vi "Main Page.vi"(8 "error in (no error)":errorcluster, 11 "Node Ptr":T1 format="%.0x") -> (0 "error out":errorcluster)   [LabVIEW 2027, in "Embedded Data Logger System Explorer.lvlib"]
uses:
  Embedded Data Logger System Explorer.lvlib
  <vilib>/NI VeriStand/Custom Device API/Custom Device Item Ref.ctl
  <vilib>/NI VeriStand/Custom Device API/Custom Device API.lvlib
  Scripting/Embedded Data Logger Scripting.lvlib
panel:
  in  "Header 2":cluster{"Section Name":string}={"Section Name"="TDMS Data Log Files"}
  in  "Remove":bool
  in  "TDMS Log Files":i32(listbox)
  in  "FIFO Depth":i32=100
  in  "Add File":bool
  in  "Header":cluster{"Section Name":string}={"Section Name"="Embedded Data Logger Settings"}
  in  "Name":string
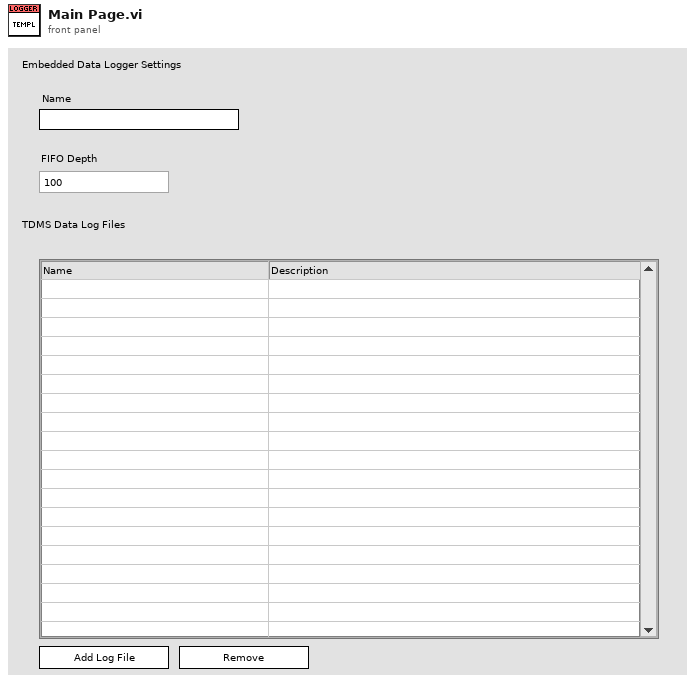
[diagram p1: front panel]
types:
  T1 = typedef "Custom Device API.lvlib/Custom Device Item Ref.ctl" = u64
  T2 = typedef "Custom Device API.lvlib/Custom Device Item Info.ctl" = cluster{"Name":string, "Is Channel":bool, "GUID":string, "Is Waveform":bool}
  T3 = typedef "Custom Device API.lvlib/Custom Device Commands.ctl" = enum16{"Default", "Item renamed", "Shutdown", "Dynamic button pressed"}
  T4 = typedef "LVRowAndColumnTypeDef.ctl" = cluster{"Row":i32, "Column":i32}
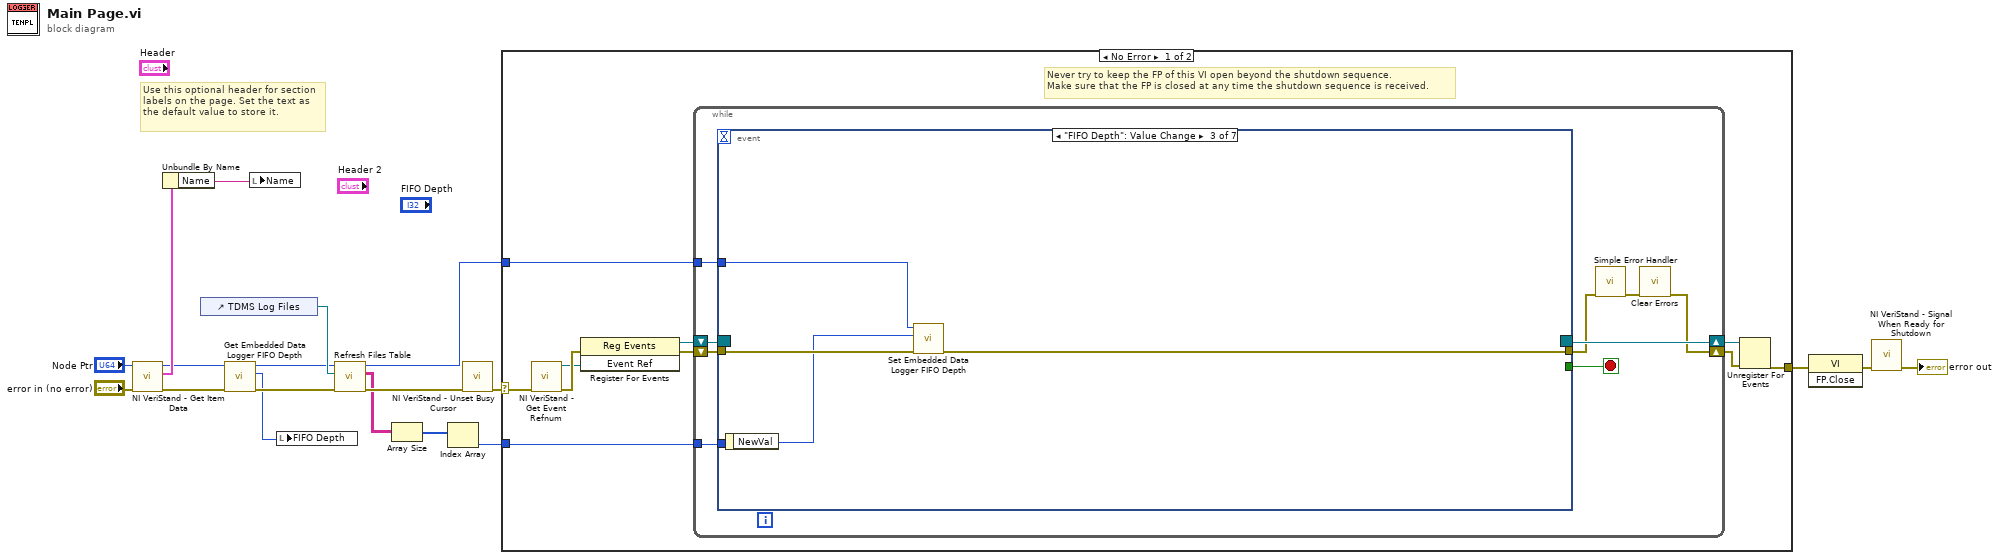
[diagram p0: block diagram]
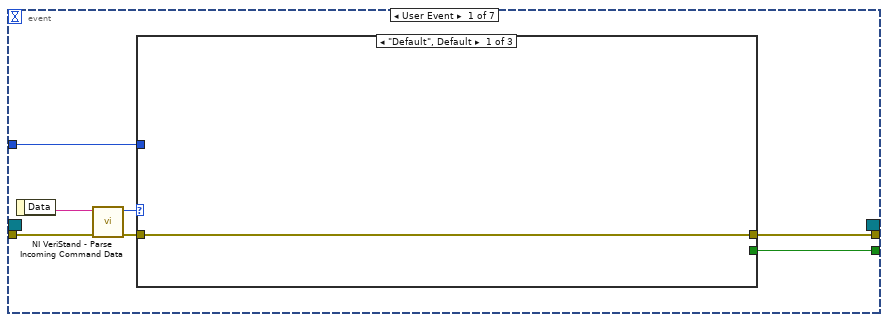
[diagram p2: hidden frame]
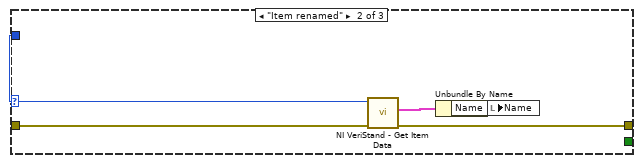
[diagram p3: hidden frame]
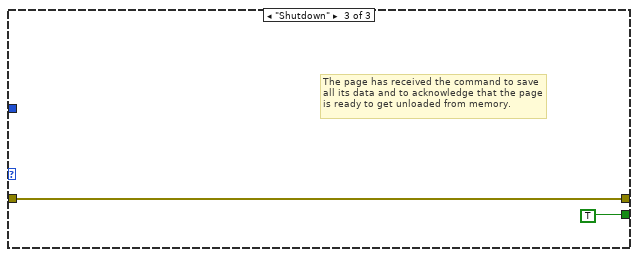
[diagram p4: hidden frame]
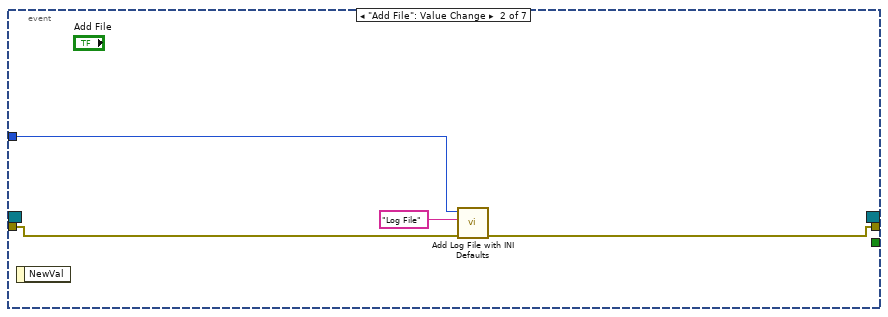
[diagram p5: hidden frame]
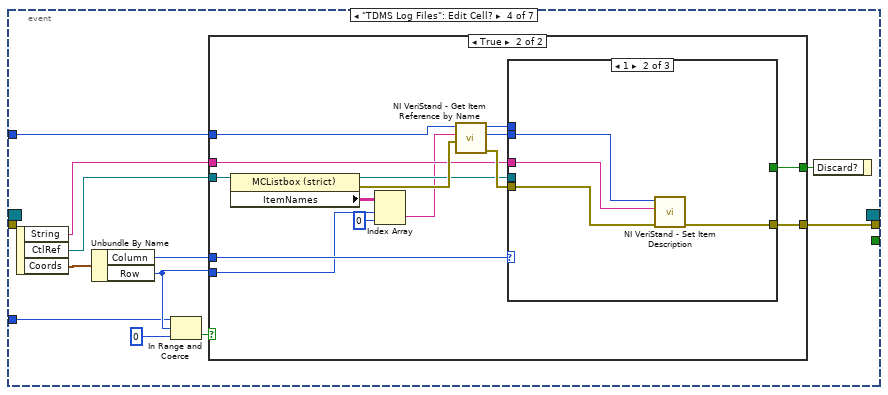
[diagram p6: hidden frame]
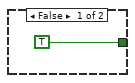
[diagram p7: hidden frame]
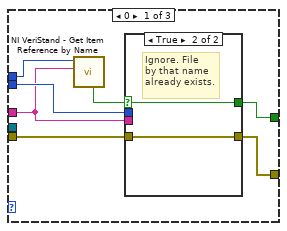
[diagram p8: hidden frame]
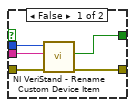
[diagram p9: hidden frame]
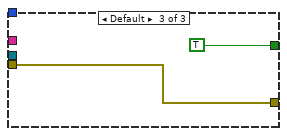
[diagram p10: hidden frame]
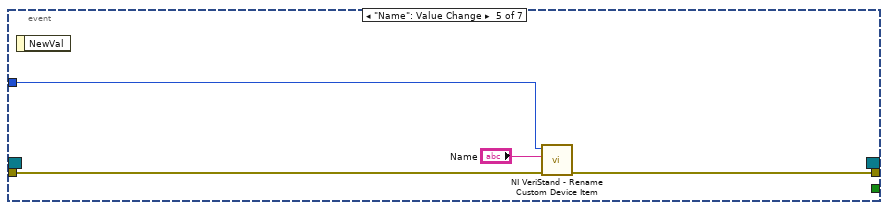
[diagram p11: hidden frame]
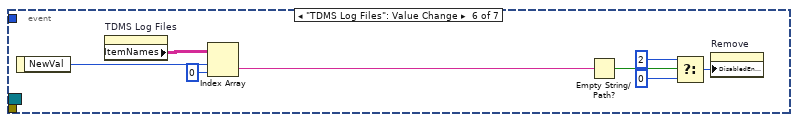
[diagram p12: hidden frame]
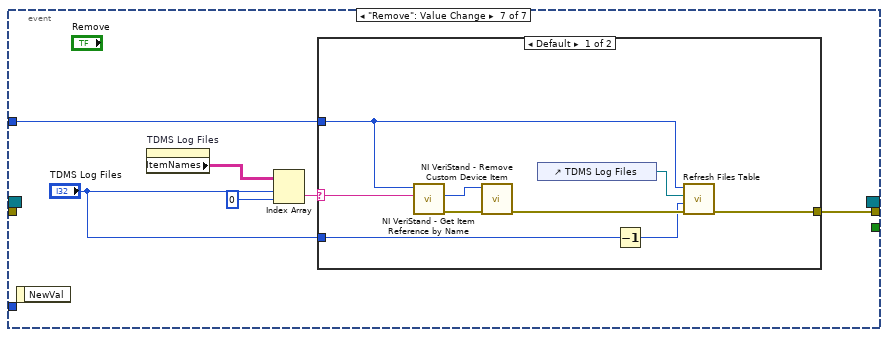
[diagram p13: hidden frame]
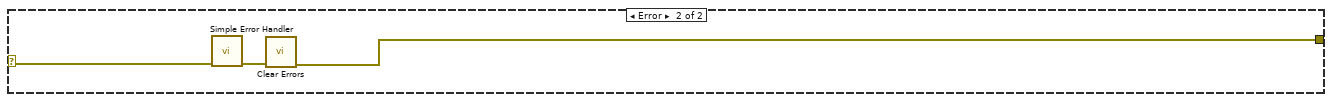
[diagram p15: hidden frame]
diagram:
  # "Use this optional header for section labels on the page. Set the text as the default value to store it."
  n1 = call <vilib>:"NI VeriStand - Get Item Data.vi"("error in (no error)"="error in (no error)", "Item Ref in"="Node Ptr") -> ("error out"=w12:errorcluster, "Item Info"=w14:T2, "Item Ref out"=w11:T1)  [unwired: 7 out]
  n2 = Unbundle By Name(w14) -> ("Name"=w13:string)
  n3 = control-ref of="TDMS Log Files"() -> (w2:refnum<vi>)
  n4 = call "Get Embedded Data Logger FIFO Depth.vi"("error in"=w12, "embedded data logger in"=w11) -> ("error out"=w19:errorcluster, "fifo depth"=w10:i32, "embedded data logger out"=w1:T1)  [unwired: 7 in]
  n5 = local write "Name"(w13) -> ()
  n6 = local write "FIFO Depth"(w10) -> ()
  n7 = call "Refresh Files Table.vi"("error in (no error)"=w19, "MulticolumnListbox in"=w2, "Section Ref in"=w1) -> ("error out"=w9:errorcluster, "Array"=w8:string[][], "Section Ref out"=w5:T1)  [unwired: 6 in]
  n8 = Array Size(array=w8) -> (size(s)=w7:i32[])
  n9 = Index Array(array=w7) -> (element=w6:i32)  [unwired: 1 in]
  n10 = call <vilib>:"NI VeriStand - Unset Busy Cursor.vi"("error in (no error)"=w9) -> ("error out"=w15:errorcluster)  [unwired: 10 out]
  n11 = case shown="No Error" w15 {
    selector: w15 -> [w21 w138]
    tunnel: [w26 w136] -> w18
    tunnel: w5 -> [w22 _]
    tunnel: w6 -> [w20 _]
    frame No Error {
      # "Never try to keep the FP of this VI open beyond the shutdown sequence.\nMake sure that the FP is closed at any time the shutdown sequence is received."
      n12 = call <vilib>:"NI VeriStand - Get Event Refnum.vi"("error in (no error)"=w21) -> ("error out"=w29:errorcluster, "Event Ref"=w25:refnum<user-event>)  [unwired: 9 out]
      n13 = register-events(error in=w29, w25) -> (reference out=w23:refnum<event-registration>, error out=w24:errorcluster)  [unwired: 1 in]
      n14 = while {
        tunnel: w22 -> [w34]
        shift-right: [w31] -> w27
        shift-left: w24 -> [w37]
        shift-right: [w38] -> w28
        shift-left: w23 -> [w36]
        tunnel: w20 -> [w30]
        stop <- w35 stop-if-true
        n15 = event shown="[2] \"FIFO Depth\": Value Change" {
          selector: w36 -> [_ _ _ _ _ _ _]
          dyn-events: [_ _ _ _ _ _ _] -> w38
          timeout: _ -> [_ _ _ _ _ _ _]
          tunnel: w37 -> [w45 w56 w61 _ w112 _ _]
          tunnel: [w41 _ _ _ _ _ _] -> w35
          tunnel: [w40 w54 w58 w68 w111 _ w123] -> w33
          tunnel: w34 -> [w39 w55 w60 w63 w110 _ w124]
          tunnel: w30 -> [_ _ _ w62 _ _ _]
          event User Event {
            n16 = event-data() -> ("Data"=w44:string)  [unwired: 1 out]
            n17 = call <vilib>:"NI VeriStand - Parse Incoming Command Data.vi"("error in (no error)"=w45, "Incoming data"=w44) -> ("error out"=w43:errorcluster, "Action"=w42:T3)  [unwired: 8 out]
            n18 = case shown="\"Default\", Default" w42 {
              tunnel: w43 -> [w46 w51 w52]
              tunnel: [_ _ TRUE] -> w41
              tunnel: [w46 w48 w52] -> w40
              tunnel: w39 -> [_ w50 _]
              frame "Default", Default {
              }
              frame "Item renamed" {
                n19 = call <vilib>:"NI VeriStand - Get Item Data.vi"("error in (no error)"=w51, "Item Ref in"=w50) -> ("error out"=w48:errorcluster, "Item Info"=w49:T2)  [unwired: 8 out]
                n20 = Unbundle By Name(w49) -> ("Name"=w47:string)
                n21 = local write "Name"(w47) -> ()
              }
              frame "Shutdown" {
                # "The page has received the command to save all its data and to acknowledge that the page is ready to get unloaded from memory."
              }
            }
          }
          event "Add File": Value Change {
            n22 = event-data() -> ()  [unwired: 2 out]
            n23 = call "Add Log File with INI Defaults.vi"("error in"=w56, "log file name"="Log File" ("Default Name"), "embedded data logger in"=w55) -> ("error out"=w54:errorcluster)  [unwired: 6 in, 2 out]
          }
          event "FIFO Depth": Value Change {
            n24 = event-data() -> ("NewVal"=w59:i32)  [unwired: 1 out]
            n25 = call "Set Embedded Data Logger FIFO Depth.vi"("error in"=w61, "fifo depth"=w59, "embedded data logger in"=w60) -> ("error out"=w58:errorcluster)  [unwired: 7 in, 1 out]
          }
          event "TDMS Log Files": Edit Cell? {
            n26 = event-data() -> ("String"=w65:string, "CtlRef"=w64:refnum<vi>, "Coords"=w66:T4)  [unwired: 1 out]
            n27 = Unbundle By Name(w66) -> ("Column"=w72:i32, "Row"=w70:i32)
            n28 = In Range and Coerce(upper limit=w62, x=w70, lower limit=0) -> (In Range?=w69:bool)  [unwired: 1 out]
            n29 = case shown="True" w69 {
              tunnel: w64 -> [_ w86]
              tunnel: [TRUE w83] -> w67
              tunnel: w65 -> [_ w81]
              tunnel: w63 -> [_ w79]
              tunnel: w70 -> [_ w78]
              tunnel: w72 -> [_ w84]
              tunnel: [_ w80] -> w68
              frame False {
              }
              frame True {
                n30 = property class="MCListbox (strict)"(reference=w86) -> (reference out=w82:refnum<vi>, error out=w88:errorcluster, "ItemNames"=w85:string[][])  [unwired: 1 in]
                n31 = Index Array(array=w85, index (row)=w78, index (col)=0 ("disabled index (col)")) -> (element=w76:string)
                n32 = call <vilib>:"NI VeriStand - Get Item Reference by Name.vi"("error in (no error)"=w88, "Item Name"=w76, "Parent Ref in"=w79) -> ("error out"=w87:errorcluster, "Item Ref"=w75:T1, "Parent Ref out"=w74:T1)  [unwired: 5 in, 1 out]
                n33 = case shown="1" w84 {
                  tunnel: [w89 _ TRUE] -> w83
                  tunnel: w75 -> [w94 w105 _]
                  tunnel: w87 -> [w95 w103 w107]
                  tunnel: w82 -> [_ _ _]
                  tunnel: w81 -> [w91 w104 _]
                  tunnel: [w93 w106 w107] -> w80
                  tunnel: w74 -> [w92 _ _]
                  frame 0 {
                    n34 = call <vilib>:"NI VeriStand - Get Item Reference by Name.vi"("Item Name"=w91, "Parent Ref in"=w92) -> ("Found"=w90:bool)  [unwired: 6 in, 3 out]
                    n35 = case shown="True" w90 {
                      selector: w90 -> [_ w101]
                      tunnel: w95 -> [w100 w102]
                      tunnel: w94 -> [w99 _]
                      tunnel: [w98 w102] -> w93
                      tunnel: w91 -> [w97 _]
                      tunnel: [w96 w101] -> w89
                      frame False {
                        n36 = call <vilib>:"NI VeriStand - Rename Custom Device Item.vi"("error in (no error)"=w100, "New Name"=w97, "Item Ref in"=w99) -> ("error out"=w98:errorcluster, "Request invalid?"=w96:bool)  [unwired: 6 in, 1 out]
                      }
                      frame True {
                        # "Ignore. File\nby that name\nalready exists."
                      }
                    }
                  }
                  frame 1 {
                    n37 = call <vilib>:"NI VeriStand - Set Item Description.vi"("error in (no error)"=w103, "Description"=w104, "Item Ref in"=w105) -> ("error out"=w106:errorcluster)  [unwired: 6 in, 2 out]
                  }
                  frame Default {
                  }
                }
              }
            }
            n38 = event-data("Discard?"=w67) -> ()  [unwired: 1 in, 1 out]
          }
          event "Name": Value Change {
            n39 = event-data() -> ()  [unwired: 2 out]
            n40 = call <vilib>:"NI VeriStand - Rename Custom Device Item.vi"("error in (no error)"=w112, "New Name"="Name", "Item Ref in"=w110) -> ("error out"=w111:errorcluster)  [unwired: 1 in, 7 out]
          }
          event "TDMS Log Files": Value Change {
            n41 = event-data() -> ("NewVal"=w113:i32)  [unwired: 1 out]
            n42 = property on="TDMS Log Files" class="MCListbox (strict)"() -> ("ItemNames"=w114:string[][])  [unwired: 2 in, 2 out]
            n43 = Index Array(array=w114, index (row)=w113, index (col)=0 ("disabled index (col)")) -> (element=w117:string)
            n44 = Empty String/Path?(string/path=w117) -> (empty?=w116:bool)
            n45 = Select(t=u8 2, s=w116, f=u8 0) -> (s? t:f=w118:u8)
            n46 = property on="Remove" class="Bool"("DisabledEnum"=w118) -> ()  [unwired: 2 in, 2 out]
          }
          event "Remove": Value Change {
            n47 = event-data() -> ()  [unwired: 2 out]
            n48 = property on="TDMS Log Files" class="MCListbox (strict)"() -> ("ItemNames"=w122:string[][])  [unwired: 2 in, 2 out]
            n49 = Index Array(array=w122, index (row)="TDMS Log Files", index (col)=0 ("disabled index (col)")) -> (element=w126:string)
            n50 = case shown="Default" w126 {
              selector: w126 -> [w134 _]
              tunnel: w124 -> [w129 _]
              tunnel: [w130 _] -> w123
              tunnel: "TDMS Log Files" -> [w127 _]
              frame Default {
                n51 = call <vilib>:"NI VeriStand - Get Item Reference by Name.vi"("Item Name"=w134, "Parent Ref in"=w129) -> ("error out"=w135:errorcluster, "Item Ref"=w133:T1)  [unwired: 6 in, 2 out]
                n52 = call <vilib>:"NI VeriStand - Remove Custom Device Item.vi"("error in (no error)"=w135, "Item Ref in"=w133) -> ("error out"=w131:errorcluster)  [unwired: 8 in, 1 out]
                n53 = control-ref of="TDMS Log Files"() -> (w132:refnum<vi>)
                n54 = Decrement(x=w127) -> (x-1=w128:i32)
                n55 = call "Refresh Files Table.vi"("error in (no error)"=w131, "Index"=w128, "MulticolumnListbox in"=w132, "Section Ref in"=w129) -> ("error out"=w130:errorcluster)  [unwired: 5 in, 2 out]
              }
              frame "" {
              }
            }
          }
        }
        n56 = call <vilib>:"Simple Error Handler.vi"("error in (no error)"=w33) -> ("error out"=w32:errorcluster)  [unwired: 1 in, 7 out]
        n57 = call <vilib>:"Clear Errors.vi"("error in (no error)"=w32) -> ("error out"=w31:errorcluster)  [unwired: 1 in, 5 out]
      }
      n58 = Unregister For Events(event registration refnum=w28, error in=w27) -> (error out=w26:errorcluster)
    }
    frame Error {
      n59 = call <vilib>:"Simple Error Handler.vi"("error in (no error)"=w138) -> ("error out"=w137:errorcluster)  [unwired: 1 in, 7 out]
      n60 = call <vilib>:"Clear Errors.vi"("error in (no error)"=w137) -> ("error out"=w136:errorcluster)  [unwired: 1 in, 5 out]
    }
  }
  n61 = invoke class="VI" method="FP.Close"(error in=w18) -> (error out=w17:errorcluster)  [unwired: 2 in, 2 out]
  n62 = call <vilib>:"NI VeriStand - Signal When Ready for Shutdown.vi"("error in (no error)"=w17) -> ("error out"=→"error out":errorcluster)  [unwired: 10 out]
